vi "wavelength to color.vi"(0 "Wavelength (380 - 780)":dbl(slide)=380.0 scale=380.0..780.0) -> (1 "Color":u32(colorbox)=4980812, 2 "Out Of Range":bool)   [LabVIEW 2021]
panel:
  # "This VI uses a straight line approximation of the RGB values in the\nvisible light spectrum according to this picture.\n\nThe algorithm consists of several straight line equations, and an straight-line approximation of fall-off of the intensities at the edge of the spectrum."
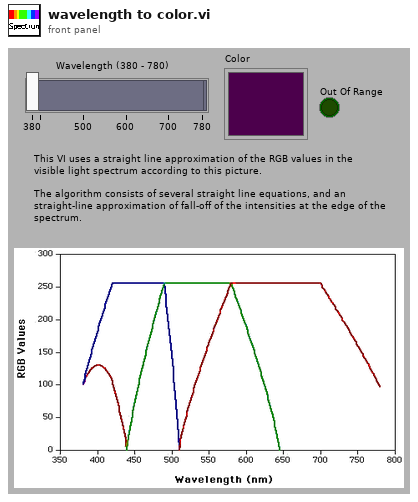
[diagram p1: front panel]
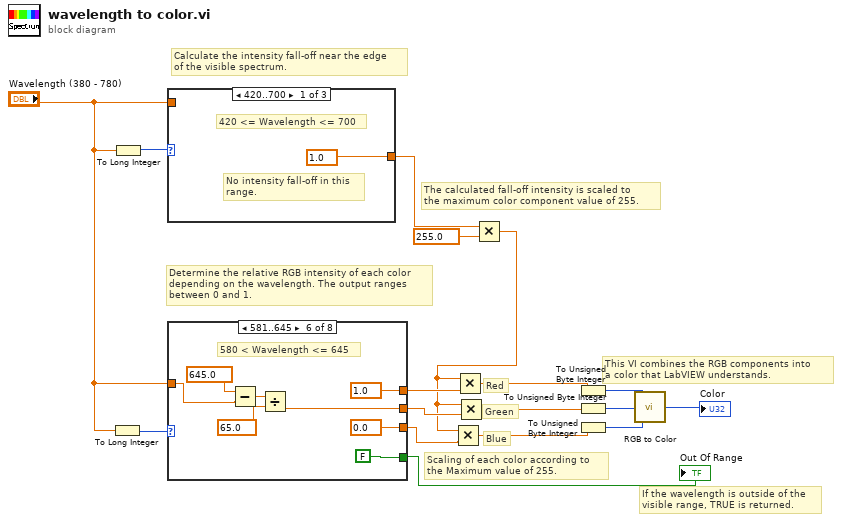
[diagram p0: block diagram]
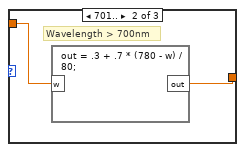
[diagram p2: hidden frame]
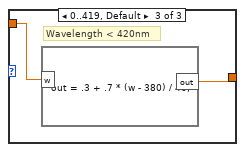
[diagram p3: hidden frame]
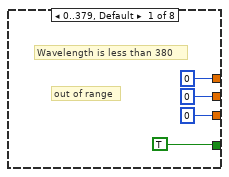
[diagram p4: hidden frame]
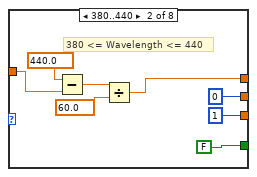
[diagram p5: hidden frame]
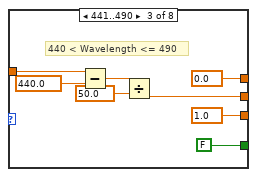
[diagram p6: hidden frame]
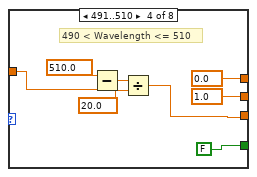
[diagram p7: hidden frame]
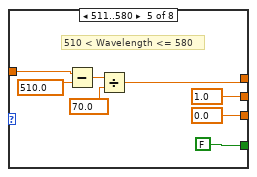
[diagram p8: hidden frame]
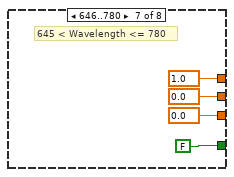
[diagram p9: hidden frame]
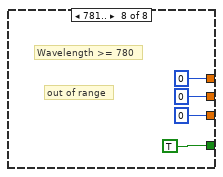
[diagram p10: hidden frame]
diagram:
  # "This VI combines the RGB components into\na color that LabVIEW understands."
  # "If the wavelength is outside of the\nvisible range, TRUE is returned."
  # "Blue"
  # "Green"
  # "Red"
  # "The calculated fall-off intensity is scaled to\nthe maximum color component value of 255."
  # "Scaling of each color according to\nthe Maximum value of 255."
  # "Determine the relative RGB intensity of each color\ndepending on the wavelength. The output ranges\nbetween 0 and 1."
  # "Calculate the intensity fall-off near the edge\nof the visible spectrum."
  n1 = To Long Integer(number="Wavelength (380 - 780)") -> (32bit integer=w3:i32)
  n2 = To Long Integer(number="Wavelength (380 - 780)") -> (32bit integer=w1:i32)
  n3 = case shown="420..700" w1 {
    tunnel: "Wavelength (380 - 780)" -> [_ w20 w21]
    tunnel: [1.0 w19 w22] -> w12
    frame 420..700 {
      # "No intensity fall-off in this\nrange."
      # "420 <= Wavelength <= 700"
    }
    frame 701.. {
      # "Wavelength > 700nm"
      n4 = formula code="out = .3 + .7 * (780 - w) / 80;"("w"=w20) -> ("out"=w19:dbl)
    }
    frame 0..419, Default {
      # "Wavelength < 420nm"
      n5 = formula code="out = .3 + .7 * (w - 380) / 40;"("w"=w21) -> ("out"=w22:dbl)
    }
  }
  n6 = case shown="581..645" w3 {
    tunnel: "Wavelength (380 - 780)" -> [_ w31 w41 w48 w57 w65 _ _]
    tunnel: [u32 0 w27 0.0 0.0 w53 1.0 1.0 u32 0] -> w10
    tunnel: [u32 0 u32 0 w37 1.0 1.0 w61 0.0 u32 0] -> w9
    tunnel: [u32 0 u32 1 1.0 w45 0.0 0.0 0.0 u32 0] -> w8
    tunnel: [TRUE FALSE FALSE FALSE FALSE FALSE FALSE TRUE] -> w17
    frame 0..379, Default {
      # "out of range"
      # "Wavelength is less than 380"
    }
    frame 380..440 {
      # "380 <= Wavelength <= 440"
      n7 = Subtract(x=440.0, y=w31) -> (x-y=w29:dbl)
      n8 = Divide(x=w29, y=60.0) -> (x/y=w27:dbl)
    }
    frame 441..490 {
      # "440 < Wavelength <= 490"
      n9 = Subtract(x=w41, y=440.0) -> (x-y=w39:dbl)
      n10 = Divide(x=w39, y=50.0) -> (x/y=w37:dbl)
    }
    frame 491..510 {
      # "490 < Wavelength <= 510"
      n11 = Subtract(x=510.0, y=w48) -> (x-y=w47:dbl)
      n12 = Divide(x=w47, y=20.0) -> (x/y=w45:dbl)
    }
    frame 511..580 {
      # "510 < Wavelength <= 580"
      n13 = Subtract(x=w57, y=510.0) -> (x-y=w55:dbl)
      n14 = Divide(x=w55, y=70.0) -> (x/y=w53:dbl)
    }
    frame 581..645 {
      # "580 < Wavelength <= 645"
      n15 = Subtract(x=645.0, y=w65) -> (x-y=w63:dbl)
      n16 = Divide(x=w63, y=65.0) -> (x/y=w61:dbl)
    }
    frame 646..780 {
      # "645 < Wavelength <= 780"
    }
    frame 781.. {
      # "out of range"
      # "Wavelength >= 780"
    }
  }
  "Out Of Range" <- w17
  n17 = Multiply(x=w12, y=255.0) -> (x*y=w4:dbl)
  n18 = Multiply(x=w4, y=w8) -> (x*y=w5:dbl)
  n19 = Multiply(x=w4, y=w10) -> (x*y=w7:dbl)
  n20 = Multiply(x=w4, y=w9) -> (x*y=w6:dbl)
  n21 = To Unsigned Byte Integer(number=w7) -> (unsigned 8bit integer=w15:u8)
  n22 = To Unsigned Byte Integer(number=w6) -> (unsigned 8bit integer=w14:u8)
  n23 = To Unsigned Byte Integer(number=w5) -> (unsigned 8bit integer=w13:u8)
  n24 = call <vilib>:"RGB to Color.vi"("B"=w13, "G"=w14, "R"=w15) -> ("Color"=→"Color":u32)
